vi "Workspace.Initialize.vi"(11 "State":T1) -> (0 "error out":errorcluster, 3 "State":T1)   [LabVIEW 2019, in "J1939 Workspace Shared.lvlib"]
uses:
  J1939 Workspace Shared.lvlib
  Types/UI.StateVariables.ctl
  <vilib>/NI VeriStand/Display Template Support/DisplayTemplateSupport.llb/enum_Display Template Handler Minimal To Widget Msg.ctl
  <vilib>/NI VeriStand/Execution/Workspace/SystemStateRegEventRef.ctl
  <vilib>/NI VeriStand/Execution/Workspace/Target State Info.ctl
  <vilib>/NI VeriStand/Execution/Workspace/Target State.ctl
  Shared/Types/Private Data.ctl
  <vilib>/NI/STM/TCP/TCP Connection Info.ctl
  <vilib>/NI/STM/SubVIs/MetaDataElement.ctl
  Shared/Types/Error Cluster.ctl
  Shared/Types/Error Types.ctl
  NationalInstruments.VeriStand.SystemStorage
  <vilib>/NI VeriStand/Display Template Support/DisplayTemplateSupport.llb/enum_Display Template Handler Minimal To Workspace.ctl
  <vilib>/NI VeriStand/Execution/Workspace/WorkspaceAPI.ctl
  NationalInstruments.VeriStand.ClientAPI
  <vilib>/NI VeriStand/Execution/Workspace/SystemStateEventRef.ctl
  Types/UI.Refs.ctl
  <vilib>/NI VeriStand/Execution/Workspace/NI_VS Workspace ExecutionAPI.lvlib
  Shared/J1939 Addon Shared.lvlib
  <vilib>/NI/STM/NI STM.lvlib
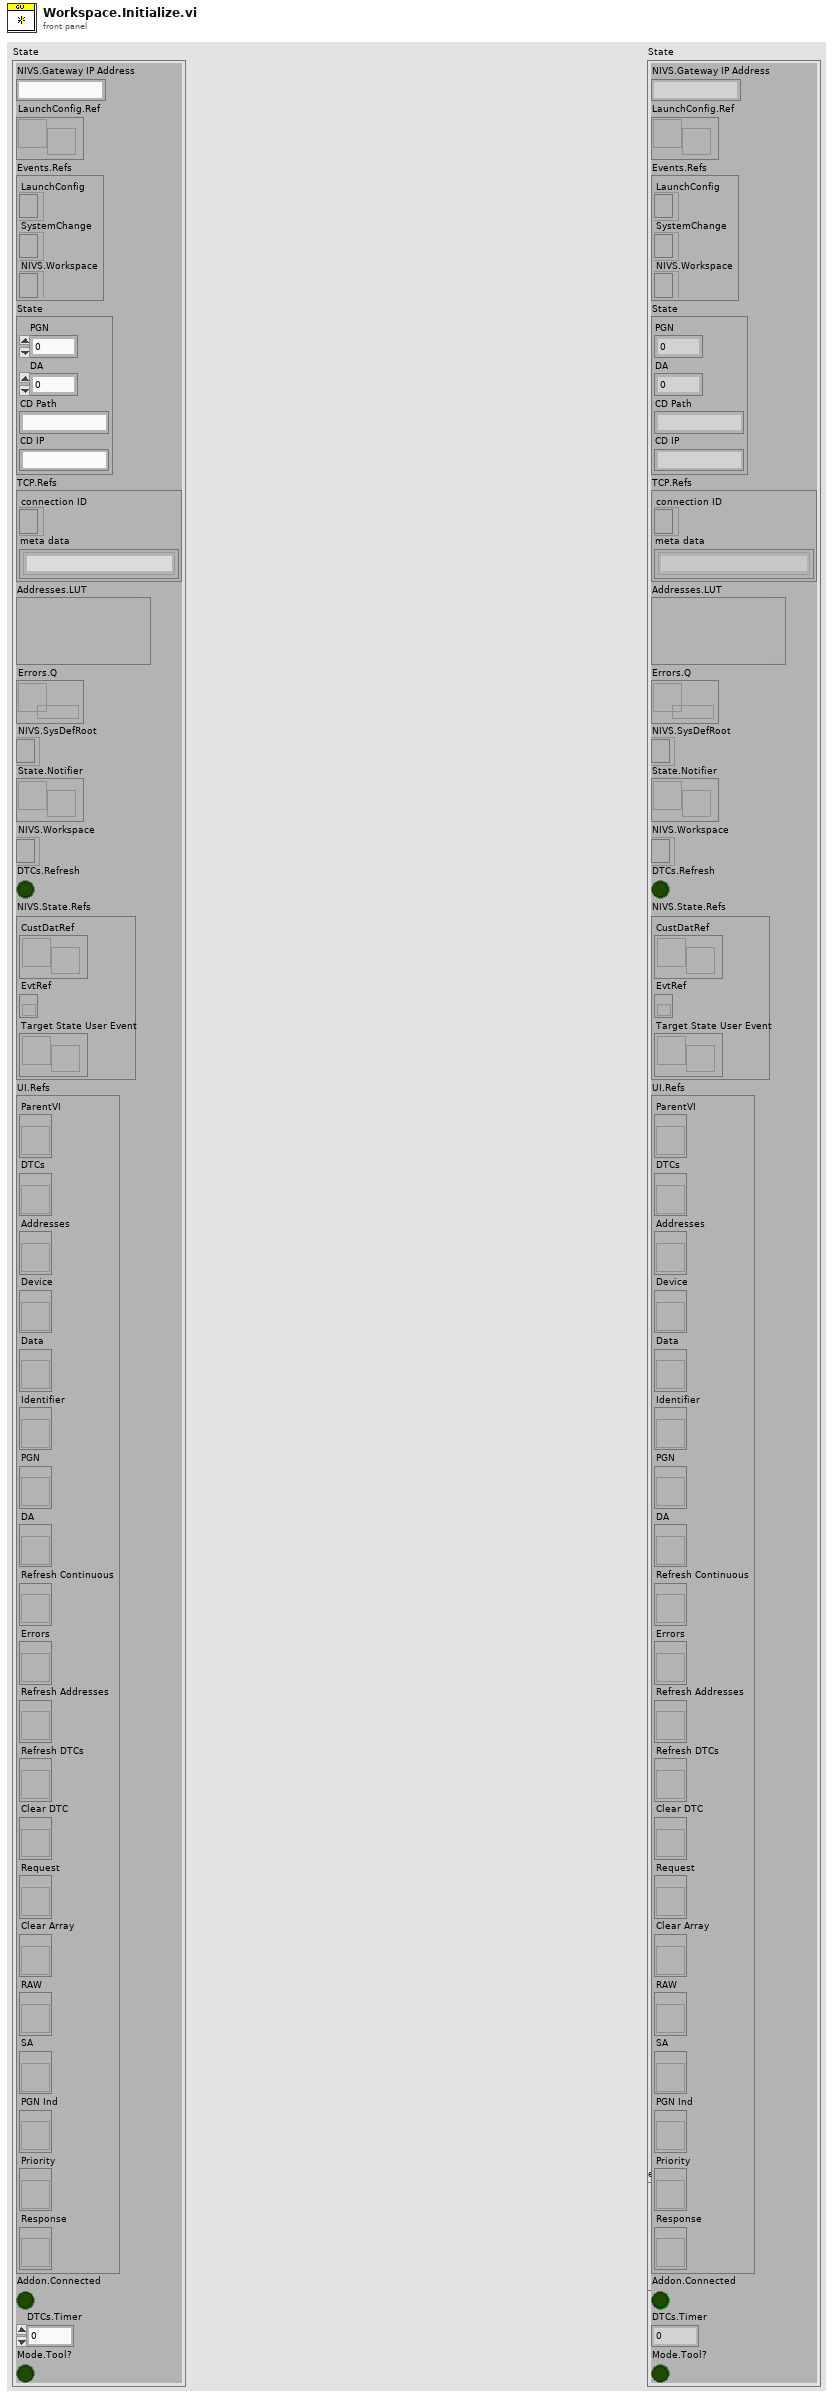
[diagram p1: front panel]
types:
  T1 = typedef "J1939 Workspace Shared.lvlib/UI.StateVariables.ctl" = cluster{"NIVS.Gateway IP Address":string, "LaunchConfig.Ref":refnum<user-event>, "Events.Refs":cluster{"LaunchConfig":refnum<event-registration>, "SystemChange":T2, "NIVS.Workspace":refnum<event-registration>}, "State":T3, "TCP.Refs":T4, "Addresses.LUT":variant, "Errors.Q":refnum<queue>, "NIVS.SysDefRoot":refnum<k24>, "State.Notifier":refnum<user-event>, "NIVS.Workspace":T6, "DTCs.Refresh":bool, "NIVS.State.Refs":T7, "UI.Refs":T8, "Addon.Connected":bool, "DTCs.Timer":u32, "Mode.Tool?":bool}
  T2 = typedef "NI_VS Workspace ExecutionAPI.lvlib/SystemStateRegEventRef.ctl" = refnum<event-registration>
  T3 = typedef "J1939 Addon Shared.lvlib/Private Data.ctl" = cluster{"PGN":u32, "DA":u8, "CD Path":string, "CD IP":string}
  T4 = typedef "NI STM.lvlib/TCP Connection Info.ctl" = cluster{"connection ID":refnum<k5>, "meta data":T5[]}
  T5 = typedef "NI STM.lvlib/MetaDataElement.ctl" = string
  T6 = typedef "NI_VS Workspace ExecutionAPI.lvlib/WorkspaceAPI.ctl" = refnum<k24>
  T7 = typedef "NI_VS Workspace ExecutionAPI.lvlib/SystemStateEventRef.ctl" = cluster{"CustDatRef":refnum<user-event>, "EvtRef":refnum<k27>, "Target State User Event":refnum<user-event>}
  T8 = typedef "J1939 Workspace Shared.lvlib/UI.Refs.ctl" = cluster{"ParentVI":refnum<vi>, "DTCs":refnum<vi>, "Addresses":refnum<vi>, "Device":refnum<vi>, "Data":refnum<vi>, "Identifier":refnum<vi>, "PGN":refnum<vi>, "DA":refnum<vi>, "Refresh Continuous":refnum<vi>, "Errors":refnum<vi>, "Refresh Addresses":refnum<vi>, "Refresh DTCs":refnum<vi>, "Clear DTC":refnum<vi>, "Request":refnum<vi>, "Clear Array":refnum<vi>, "RAW":refnum<vi>, "SA":refnum<vi>, "PGN Ind":refnum<vi>, "Priority":refnum<vi>, "Response":refnum<vi>}
  T9 = typedef "J1939 Addon Shared.lvlib/Error Cluster.ctl" = cluster{"error out":errorcluster, "Enum":T10, "Address":u8, "Timestamp":timestamp}
  T10 = typedef "J1939 Addon Shared.lvlib/Error Types.ctl" = enum16{"Request", "RAW Generation", "Clear Active DTCs", "Clear Previous DTCs", "Addresses", "TLAs", "Get Active DTCs", "Get Previous DTCs", "TCP Connection"}
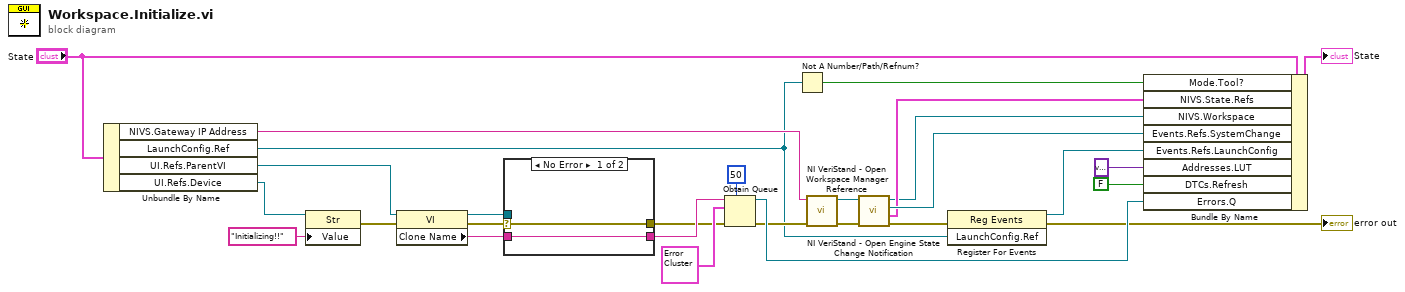
[diagram p0: block diagram]
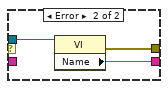
[diagram p2: hidden frame]
diagram:
  n1 = Unbundle By Name("State") -> ("NIVS.Gateway IP Address"=w16:string, "LaunchConfig.Ref"=w2:refnum<user-event>, "UI.Refs.ParentVI"=w12:refnum<vi>, "UI.Refs.Device"=w4:refnum<vi>)
  n2 = property class="Str"(reference=w4, "Value"="Initializing!!") -> (error out=w5:errorcluster)  [unwired: 1 in, 1 out]
  n3 = property class="VI"(reference=w12, error in=w5) -> (reference out=w9:refnum<vi>, error out=w10:errorcluster, "Clone Name"=w6:string)
  n4 = case shown="No Error" w10 {
    selector: w10 -> [w29 _]
    tunnel: w9 -> [_ w33]
    tunnel: [w30 w32] -> w8
    tunnel: [w29 w31] -> w7
    tunnel: w6 -> [w30 _]
    frame No Error {
    }
    frame Error {
      n5 = property class="VI"(reference=w33) -> (error out=w31:errorcluster, "Name"=w32:string)  [unwired: 1 in, 1 out]
    }
  }
  n6 = Obtain Queue(max queue size (-1, unlimited)=50, name (unnamed)=w8, element data type=T9 {"error out"={"status"=FALSE, "code"=0, "source"=""}, "Enum"=enum."Request", "Address"=0, "Timestamp"=timestamp(0 s since 1904-01-01)} ("Error Cluster"), error in (no error)=w7) -> (queue out=w28:refnum<queue>, error out=w11:errorcluster)  [unwired: 1 in, 1 out]
  n7 = Not A Number/Path/Refnum?(number/path/refnum=w2) -> (NaN/Path/Refnum?=w1:bool)
  n8 = call <vilib>:"NI VeriStand - Open Workspace Manager Reference.vi"("error in (no error)"=w11, "Gateway IP Address (\"\": localhost)"=w16) -> ("error out"=w14:errorcluster, "WorkspaceManager"=w13:T6)  [unwired: 8 in]
  n9 = call <vilib>:"NI VeriStand - Open Engine State Change Notification.vi"("error in (no error)"=w14, "WorkspaceManager in"=w13) -> ("error out"=w15:errorcluster, "SystemStateRefs"=w24:T7, "SystemChangeEventRef"=w26:T2, "WorkspaceManager out"=w18:T6)  [unwired: 6 in]
  n10 = register-events(error in=w15, w2) -> (reference out=w25:refnum<event-registration>, error out=→"error out":errorcluster)  [unwired: 1 in]
  n11 = Bundle By Name(cluster="State", "Mode.Tool?"=w1, "NIVS.State.Refs"=w24, "NIVS.Workspace"=w18, "Events.Refs.SystemChange"=w26, "Events.Refs.LaunchConfig"=w25, "Addresses.LUT"=variant ("Addresses"), "DTCs.Refresh"=FALSE, "Errors.Q"=w28) -> (→"State":T1)
